vi "finishUp.vi"(8 "error in (no error)":errorcluster, 11 "Rf_Ramp_Action in":refnum<class "Rf_Ramp_Action.lvclass">) -> (0 "error out":errorcluster, 3 "Rf_Ramp_Action out":refnum<class "Rf_Ramp_Action.lvclass">)   [LabVIEW 2009, in "Views.lvlib" / "ScriptEditor.lvlib" / "Rf_Ramp_Action.lvclass"]
uses:
  Rf_Ramp_Action.lvclass
  Rf_Ramp_Action.lvclass/Rf_Ramp_Action.ctl
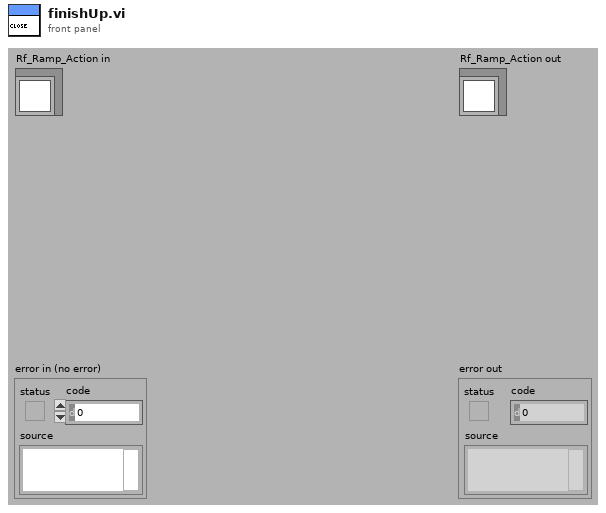
[diagram p1: front panel]
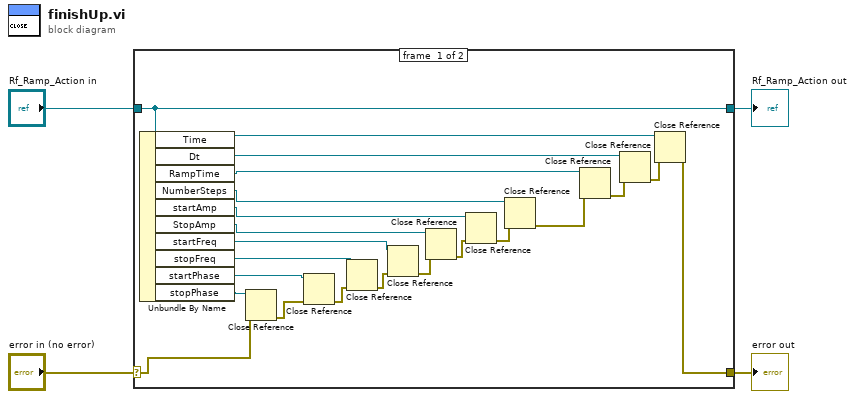
[diagram p0: block diagram]
diagram:
  n1 = case shown="No Error" "error in (no error)" {
    selector: "error in (no error)" -> [w6 w28]
    tunnel: [w7 w28] -> w3
    tunnel: [w19 w27] -> w1
    tunnel: "Rf_Ramp_Action in" -> [w19 w27]
    frame #0 {
      n2 = Unbundle By Name(w19) -> ("Time"=w9:refnum<vi>, "Dt"=w10:refnum<vi>, "RampTime"=w11:refnum<vi>, "NumberSteps"=w12:refnum<vi>, "startAmp"=w13:refnum<vi>, "StopAmp"=w14:refnum<vi>, "startFreq"=w15:refnum<vi>, "stopFreq"=w16:refnum<vi>, "startPhase"=w17:refnum<vi>, "stopPhase"=w18:refnum<vi>)
      n3 = Close Reference(reference=w18, error in (no error)=w6) -> (error out=w20:errorcluster)
      n4 = Close Reference(reference=w17, error in (no error)=w20) -> (error out=w21:errorcluster)
      n5 = Close Reference(reference=w16, error in (no error)=w21) -> (error out=w22:errorcluster)
      n6 = Close Reference(reference=w15, error in (no error)=w22) -> (error out=w23:errorcluster)
      n7 = Close Reference(reference=w14, error in (no error)=w23) -> (error out=w24:errorcluster)
      n8 = Close Reference(reference=w13, error in (no error)=w24) -> (error out=w25:errorcluster)
      n9 = Close Reference(reference=w12, error in (no error)=w25) -> (error out=w5:errorcluster)
      n10 = Close Reference(reference=w11, error in (no error)=w5) -> (error out=w26:errorcluster)
      n11 = Close Reference(reference=w10, error in (no error)=w26) -> (error out=w8:errorcluster)
      n12 = Close Reference(reference=w9, error in (no error)=w8) -> (error out=w7:errorcluster)
    }
    frame #1 {
    }
  }
  "error out" <- w3
  "Rf_Ramp_Action out" <- w1
